vi "Init Lockin.vi"(8 "error in (no error)":errorcluster, 11 "Red Pitaya Digitizer in":refnum<class "Red Pitaya Digitizer.lvclass">) -> (0 "error out":errorcluster, 3 "Red Pitaya Digitizer out":refnum<class "Red Pitaya Digitizer.lvclass">)   [LabVIEW 2024, in "Red Pitaya Digitizer.lvclass"]
uses:
  Red Pitaya Digitizer.lvclass
  RP Core/RP Instrument/RP Instrument.lvclass
  Red Pitaya Digitizer.lvclass/Red Pitaya Digitizer.ctl
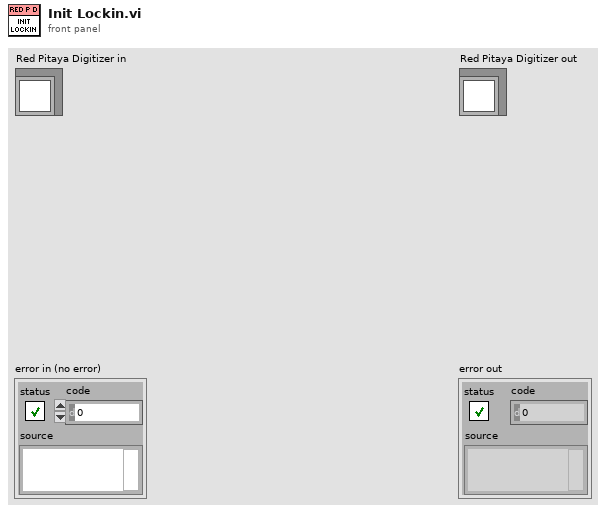
[diagram p1: front panel]
types:
  T1 = typedef "Lockin Digitizer Configuration.ctl" = cluster{"Post-trigger delay":dbl, "Post-trigger duration":dbl, "Rate":dbl, "Ranges":dbl[], "Re-name channels":string[], "Active channels":string, "External\nclock":bool, "Monitor time\nconstant":dbl, "Sync":bool, "Lock-in input channel phases":dbl[], "Output channels configuration":T2[]}
  T2 = typedef "Output Channel Configuration.ctl" = cluster{"Input channels":string, "Frequency":dbl, "Output amplitude":dbl, "Output channel number":i32}
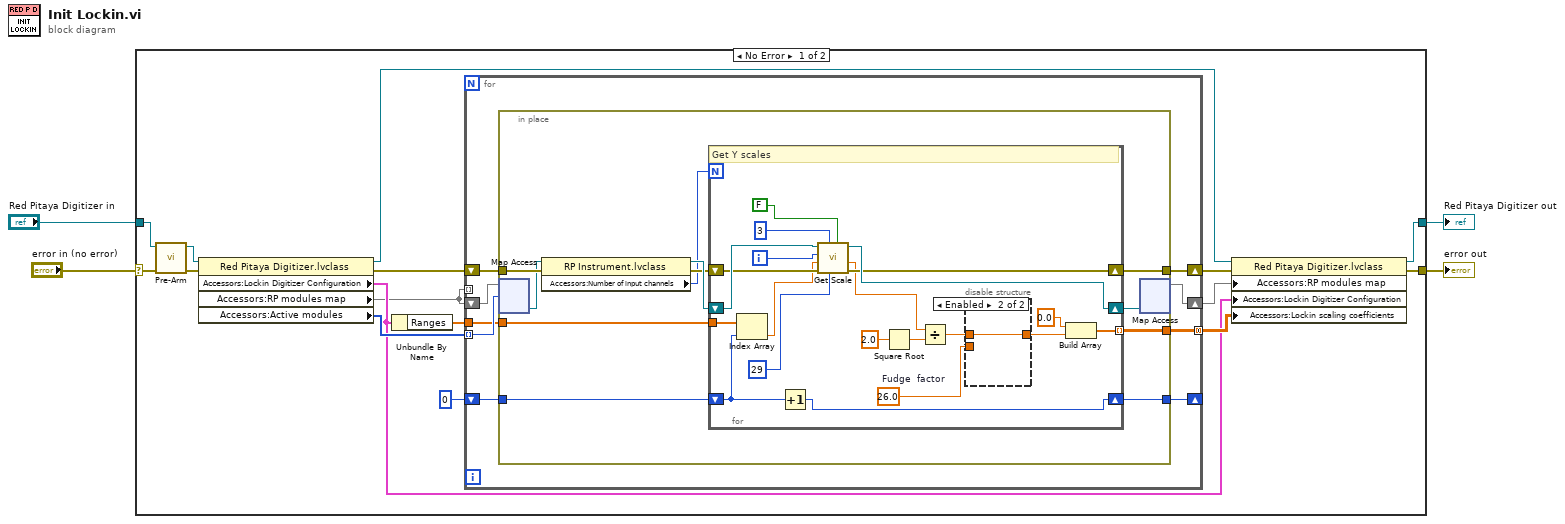
[diagram p0: block diagram]
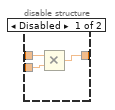
[diagram p2: hidden frame]
diagram:
  n1 = case shown="No Error" "error in (no error)" {
    selector: "error in (no error)" -> [w19 w66]
    tunnel: [w14 w66] -> w3
    tunnel: [w15 w65] -> w1
    tunnel: "Red Pitaya Digitizer in" -> [w20 w65]
    frame No Error {
      n2 = call-dynamic "Pre-Arm.vi"("error in (no error)"=w19, "Red Pitaya Digitizer in"=w20) -> ("error out"=w17:errorcluster, "Red Pitaya Digitizer out"=w18:refnum<class "Red Pitaya Digitizer.lvclass">)  [unwired: 8 in]
      n3 = property class="Red Pitaya Digitizer.lvclass"(reference=w18, error in=w17) -> (reference out=w16:refnum<class "Red Pitaya Digitizer.lvclass">, error out=w12:errorcluster, "Accessors:Lockin Digitizer Configuration"=w9:T1, "Accessors:RP modules map "=w8:map{i32, refnum<class "RP Instrument.lvclass">}, "Accessors:Active modules"=w10:i32[])
      n4 = Unbundle By Name(w9) -> ("Ranges"=w6:dbl[])
      n5 = for {
        shift-right: [w26] -> w13
        shift-left: w12 -> [w27]
        tunnel: [w25] -> w11 mode=concatenating
        tunnel: w8 -> [_] mode=indexing
        tunnel: w10 -> [w28] mode=indexing
        shift-right: [w21] -> w5
        shift-left: w8 -> [w29]
        shift-right: [w22] -> _
        shift-left: 0 -> [w23]
        tunnel: w6 -> [w24]
        n6 = in-place {
          in-place-border: w27 -> [w40]
          in-place-border: [w38] -> w26
          in-place-border: [w37] -> w25
          in-place-border: w24 -> [w34]
          in-place-border: w23 -> [w33]
          in-place-border: [w32] -> w22
          n7 = in-place-map #1(w29, w28) -> (w39:refnum<class "RP Instrument.lvclass">)  [unwired: 1 in, 1 out]
          n8 = property class="RP Instrument.lvclass"(reference=w39, error in=w40) -> (reference out=w36:refnum<class "RP Instrument.lvclass">, error out=w35:errorcluster, "Accessors:Number of input channels"=w30:i32)
          n9 = for {
            N: w30 -> [_]
            shift-right: [w58] -> w31
            shift-left: w36 -> [w60]
            shift-right: [w57] -> w38
            shift-left: w35 -> [w59]
            tunnel: [w53] -> w37 mode=indexing
            tunnel: w34 -> [w44]
            shift-right: [w42] -> w32
            shift-left: w33 -> [w43]
            i -> [w55]
            w46 = 26.0  # Fudge  factor
            # "Get Y scales"
            n10 = Index Array(array=w44, index=w43) -> (element=w41:dbl)
            n11 = Increment(x=w43) -> (x+1=w42:i32)
            n12 = call-dynamic "Get Scale.vi"("Read calibration"=FALSE, "Signal bits"=29, "Number of stages"=3, "error in (no error)"=w59, "Range"=w41, "Channel"=w55, "RP Instrument in"=w60) -> ("error out"=w57:errorcluster, "slope"=w50:dbl, "RP Instrument out"=w58:refnum<class "RP Instrument.lvclass">)  [unwired: 2 out]
            n13 = Square Root(x=2.0) -> (sqrt(x)=w51:dbl)
            n14 = Divide(x=w50, y=w51) -> (x/y=w49:dbl)
            n15 = disable-structure shown="Enabled" {
              disable-tunnel: w49 -> [w63 w64]
              disable-tunnel: [w62 w64] -> w47
              disable-tunnel: w46 -> [w61 _]
              frame Disabled {
                n16 = Multiply(x=w63, y=w61) -> (x*y=w62:dbl)
              }
              frame Enabled {
              }
            }
            n17 = Build Array(0.0 ("element"), w47) -> (w53:dbl[])
          }
          n18 = in-place-map #1(w31) -> (w21:map{i32, refnum<class "RP Instrument.lvclass">})  [unwired: 1 in, 2 out]
        }
      }
      n19 = property class="Red Pitaya Digitizer.lvclass"(reference=w16, error in=w13, "Accessors:RP modules map "=w5, "Accessors:Lockin Digitizer Configuration"=w9, "Accessors:Lockin scaling coefficients"=w11) -> (reference out=w15:refnum<class "Red Pitaya Digitizer.lvclass">, error out=w14:errorcluster)
    }
    frame Error {
    }
  }
  "error out" <- w3
  "Red Pitaya Digitizer out" <- w1
